vi "Day13-grow_and_set_array.vi"(9 "row":i32, 10 "column":i32, 11 "Array in":bool[][](array[boolean])) -> (3 "Array out":bool[][](array[boolean]))   [LabVIEW 2021]
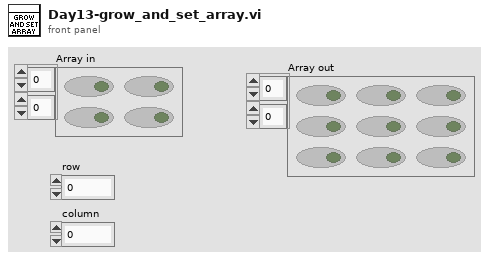
[diagram p1: front panel]
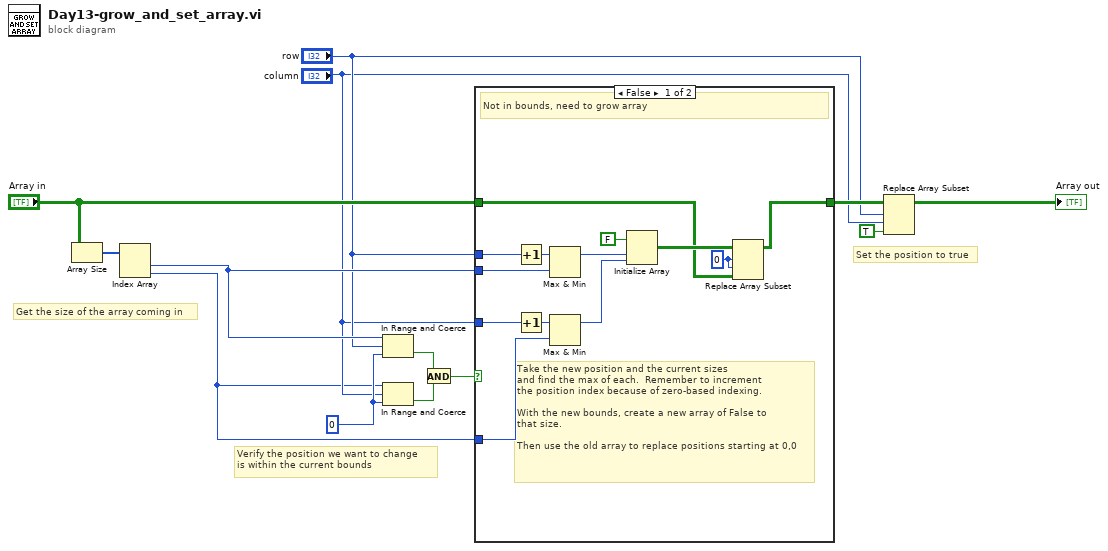
[diagram p0: block diagram]
diagram:
  w11 = 0 ("lower limit")
  # "Set the position to true"
  # "Verify the position we want to change\nis within the current bounds"
  # "Get the size of the array coming in"
  n1 = Array Size(array="Array in") -> (size(s)=w12:i32[])
  n2 = Index Array(array=w12) -> (element #1=w4:i32, element #2=w1:i32)  [unwired: 2 in]
  n3 = In Range and Coerce(upper limit=w4, x="row", lower limit=w11) -> (In Range?=w10:bool)  [unwired: 1 out]
  n4 = In Range and Coerce(upper limit=w1, x="column", lower limit=w11) -> (In Range?=w9:bool)  [unwired: 1 out]
  n5 = And(x=w10, y=w9) -> (x .and. y?=w7:bool)
  n6 = case shown="False" w7 {
    tunnel: "Array in" -> [w16 w27]
    tunnel: [w14 w27] -> w5
    tunnel: "row" -> [w25 _]
    tunnel: w4 -> [w24 _]
    tunnel: "column" -> [w20 _]
    tunnel: w1 -> [w19 _]
    frame False {
      w15 = 0 ("index (row)")
      # "Take the new position and the current sizes\nand find the max of each.  Remember to increment\nthe position index because of zero-based indexing.\n\nWith the new bounds, create a new array of False to\nthat size.\n\nThen use the old array to replace positions starting at 0,0"
      # "Not in bounds, need to grow array"
      n7 = Increment(x=w25) -> (x+1=w22:i32)
      n8 = Increment(x=w20) -> (x+1=w21:i32)
      n9 = Max & Min(x=w22, y=w24) -> (max(x,y)=w23:i32)  [unwired: 1 out]
      n10 = Max & Min(x=w21, y=w19) -> (max(x,y)=w18:i32)  [unwired: 1 out]
      n11 = Initialize Array(FALSE, w23, w18) -> (w17:bool[][])
      n12 = Replace Array Subset(array=w17, new element=w16, index (row)=w15, index (col)=w15) -> (w14:bool[][])
    }
    frame True {
      # "Within bounds, do nothing"
    }
  }
  n13 = Replace Array Subset(array=w5, new element=TRUE ("new element/subarray"), index (row)="row", index (col)="column") -> (→"Array out":bool[][])
